vi "Display Setup.vi"(8 "error in (no error)":errorcluster, 10 "Diplay":T1, 11 "Enum":T2) -> (0 "error out":errorcluster)   [LabVIEW 2015]
uses:
  Blink Rate.ctl
  Display.ctl
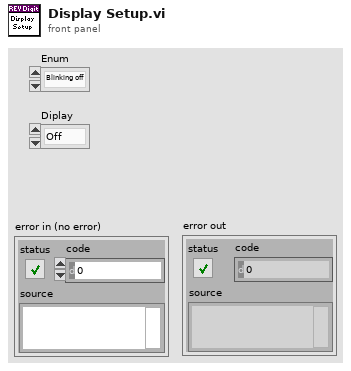
[diagram p1: front panel]
types:
  T1 = typedef "Display.ctl" = enum16{"Off", "On"}
  T2 = typedef "Blink Rate.ctl" = enum16{"Blinking off", "2 Hz", "1 Hz", "0.5 Hz"}
  T3 = typedef "WPI_I2CDevRef.ctl" = cluster{"DevStatus":errorcluster, "Device Address":u8, "Handle":i32, "I2C Bus":T4}
  T4 = typedef "i2c_bus.ctl" = enum16{"I2C On-Board", "I2C MXP", "Invalid"}
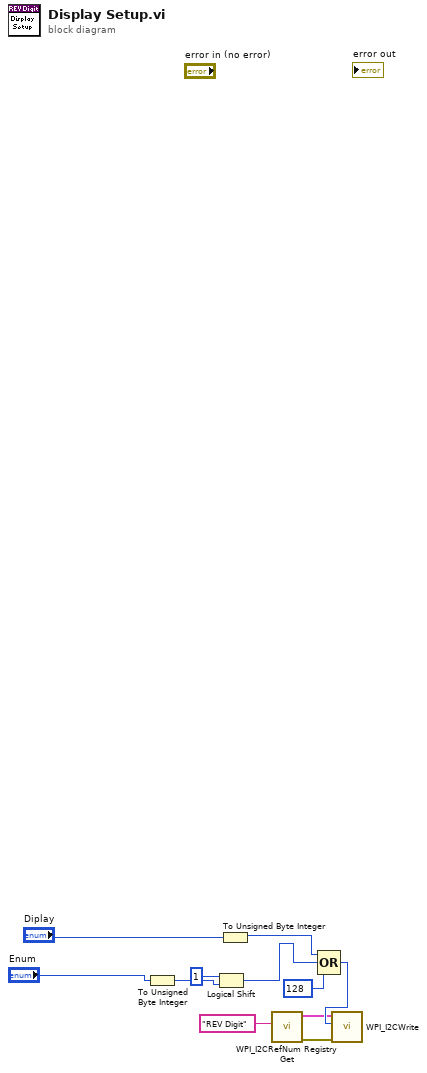
[diagram p0: block diagram]
diagram:
  n1 = To Unsigned Byte Integer(number="Enum") -> (unsigned 8bit integer=w6:u8)
  n2 = Logical Shift(y=i16 1, x=w6) -> (x << y=w10:u8)
  n3 = To Unsigned Byte Integer(number="Diplay") -> (unsigned 8bit integer=w9:u8)
  n4 = call <vilib>:"WPI_I2CRefNum Registry Get.vi"("refnum name"="REV Digit") -> ("error out"=w1:errorcluster, "I2CDevRef"=w2:T3)  [unwired: 9 in]
  n5 = Compound Arithmetic op=OR(w9, w10, u8 128 ("Device Address")) -> (w8:u8)
  n6 = call <vilib>:"WPI_I2CWrite.vi"("error in (no error)"=w1, "I2CRegister"=w8, "I2CDevRef"=w2) -> ()  [unwired: 7 in, 2 out]
